vi "save the osc screenshot.vi"(8 "Start Test_Time":string, 9 "Data in":variant, 10 "Waveform Graph Cal":waveform(dbl)(graph)) -> ()   [LabVIEW 2016]
uses:
  Global Variables/Pacemaker ASIC Test_Config Globals.vi
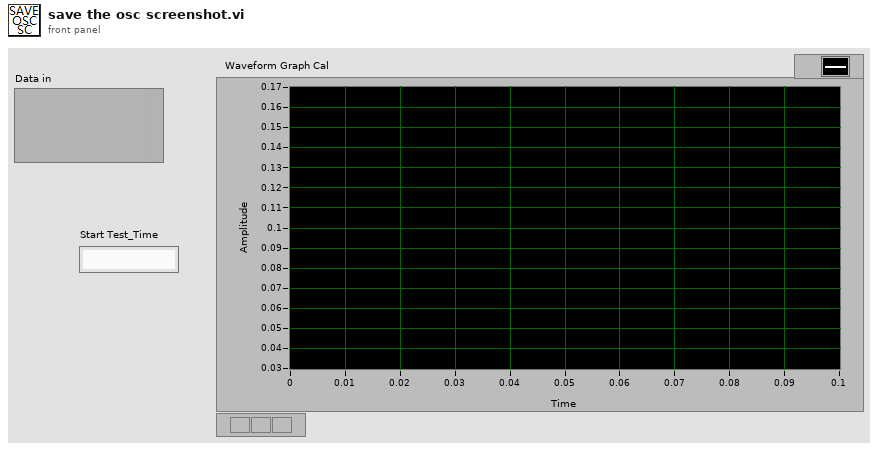
[diagram p1: front panel]
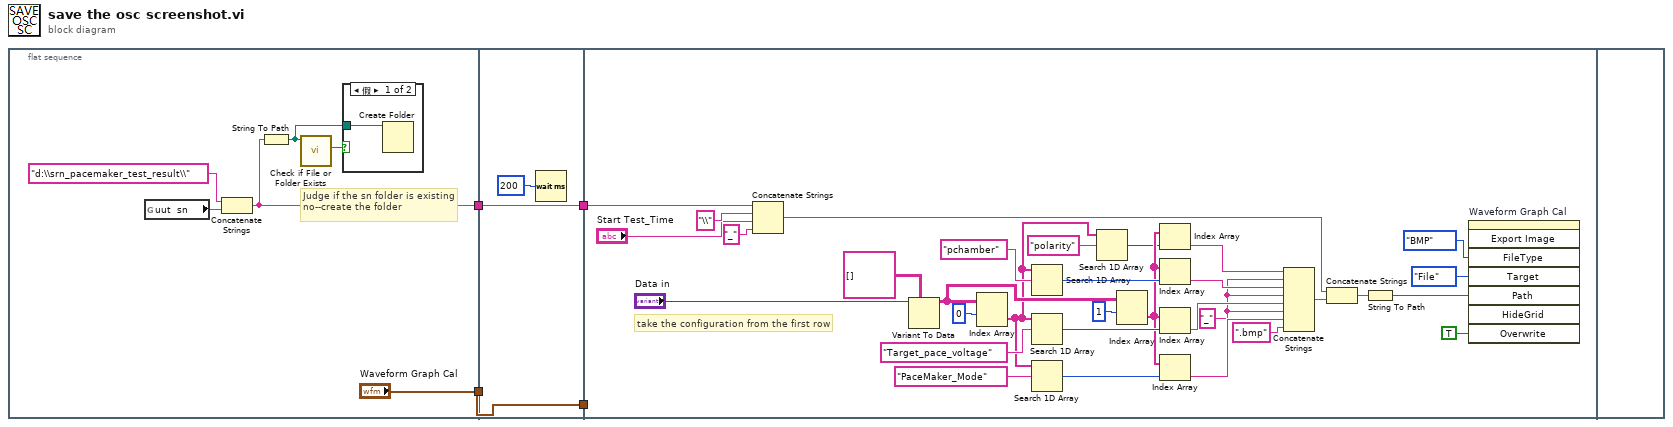
[diagram p0: block diagram]
diagram:
  n1 = flat-sequence {
    tunnel: [w6] -> w4
    tunnel: ["Waveform Graph Cal"] -> w2
    tunnel: w4 -> [w14]
    tunnel: [w14] -> w3
    tunnel: w2 -> [w13]
    tunnel: [w13] -> w1
    tunnel: w3 -> [w33]
    tunnel: w1 -> [_]
    frame #0 {
      # "Judge if the sn folder is existing\nno--create the folder"
      n2 = global read "Pacemaker ASIC Test_Config Globals.vi" "uut  sn"() -> (w10:string)
      n3 = Concatenate Strings("d:\\srn_pacemaker_test_result\\", w10) -> (w6:string)
      n4 = String To Path(string=w6) -> (path=w7:path)
      n5 = call <vilib>:"Check if File or Folder Exists.vi"("path"=w7) -> ("file or folder exists?"=w8:bool)  [unwired: 8 in, 2 out]
      n6 = case shown="假" w8 {
        tunnel: w7 -> [w11 _]
        frame False {
          n7 = Create Folder(path (use dialog)=w11) -> ()  [unwired: 2 in, 3 out]
        }
        frame True {
        }
      }
    }
    frame #1 {
      n8 = Wait (ms)(milliseconds to wait=u32 200 ("等待时间（毫秒）")) -> ()  [unwired: 1 out]
    }
    frame #2 {
      w19 = "_" ("字符串")
      # "take the configuration from the first row"
      n9 = Concatenate Strings(w33, "\\" ("字符串"), "Start Test_Time", "_" ("字符串")) -> (w29:string)
      n10 = Variant To Data(type=string[][] [], Variant="Data in") -> (data=w41:string[][])  [unwired: 1 in, 1 out]
      n11 = Index Array(array=w41, index (row)=0 ("索引 (行)")) -> (element=w24:string[])  [unwired: 1 in]
      n12 = Search 1D Array(1D array=w24, element="pchamber" ("元素")) -> (index of element=w37:i32)  [unwired: 1 in]
      n13 = Search 1D Array(1D array=w24, element="Target_pace_voltage" ("元素")) -> (index of element=w36:i32)  [unwired: 1 in]
      n14 = Search 1D Array(1D array=w24, element="PaceMaker_Mode" ("元素")) -> (index of element=w38:i32)  [unwired: 1 in]
      n15 = Search 1D Array(1D array=w24, element="polarity" ("元素")) -> (index of element=w21:i32)  [unwired: 1 in]
      n16 = Index Array(array=w41, index (row)=1 ("索引 (行)")) -> (element=w22:string[])  [unwired: 1 in]
      n17 = Index Array(array=w22, index=w21) -> (element=w20:string)
      n18 = Index Array(array=w22, index=w37) -> (element=w26:string)
      n19 = Index Array(array=w22, index=w36) -> (element=w25:string)
      n20 = Index Array(array=w22, index=w38) -> (element=w35:string)
      n21 = Concatenate Strings(w20, w19, w26, w19, w25, w19, w35, ".bmp" ("字符串")) -> (w28:string)
      n22 = Concatenate Strings(w29, w28) -> (w27:string)
      n23 = String To Path(string=w27) -> (path=w16:path)
      n24 = invoke on="Waveform Graph Cal" class="WFGraph (严格)" method="Export Image"("FileType"=enum32{"BMP", "EPS", "EMF", "PICT"}."BMP" ("文件类型"), "Target"=enum32{"File", "Clipboard"}."File" ("目标"), "Path"=w16, "Overwrite"=TRUE ("始终覆盖")) -> ()  [unwired: 4 in, 8 out]
    }
    frame #3 {
    }
  }
